vi "Run.vi"(8 "error in (no error)":errorcluster, 11 "C37.118 Sim in":refnum<class "C37.118 Sim.lvclass">) -> (0 "error out":errorcluster, 1 "DataValid":bool, 2 "clSensorData":T1, 3 "C37.118 Sim out":refnum<class "C37.118 Sim.lvclass">)   [LabVIEW 2018, in "SensorPlugins.lvlib" / "C37.118 Sim.lvclass"]
uses:
  C37.118 Sim.lvclass
  C:/projects/ICDAS/NistPluggableModules/Sensor/SensorPlugins/PmuBaseClass/PmuBase.lvclass
  SensorShared/clSensorData.ctl
  PmuBaseClass/PmuBase.lvclass/PmuBase.ctl
  PmuBaseClass/Accessors/Read PmuDataArray.vi
  PmuBaseClass/Accessors/Read PmuConfig.vi
  PmuBaseClass/Accessors/Write PmuDataArray.vi
  SensorShared/SensorShared.lvlib
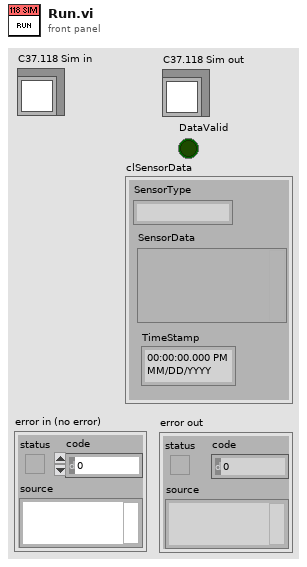
[diagram p1: front panel]
types:
  T1 = typedef "SensorShared.lvlib/clSensorData.ctl" = cluster{"SensorType":string, "SensorData":variant, "TimeStamp":timestamp}
  T2 = typedef "SensorPlugins.lvlib/PmuBase.lvclass/PmuData.ctl" = cluster{"Timestamp":dbl, "Synx":cdb[], "Freq":dbl, "ROCOF":dbl, "ID":i16}
  T3 = typedef "SensorPlugins.lvlib/PmuBase.lvclass/PmuConfig.ctl" = cluster{"Class":enum16{"M", "P"}, "Fs":i32, "F0":i32, "FSamp":i32, "SettlingTime":dbl, "T0":ext}
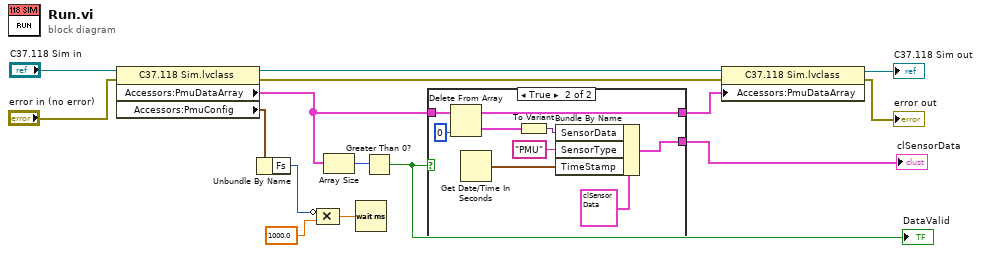
[diagram p0: block diagram]
diagram:
  n1 = property class="C37.118 Sim.lvclass"(reference="C37.118 Sim in", error in="error in (no error)") -> (reference out=w12:refnum<class "C37.118 Sim.lvclass">, error out=w11:errorcluster, "Accessors:PmuDataArray"=w5:T2[], "Accessors:PmuConfig"=w2:T3)
  n2 = Unbundle By Name(w2) -> ("Fs"=w1:i32)
  n3 = Compound Arithmetic op=MULTIPLY(invert w1, 1000.0 ("y")) -> (w8:dbl)
  n4 = Array Size(array=w5) -> (size(s)=w4:i32)
  n5 = Wait (ms)(milliseconds to wait=w8) -> ()  [unwired: 1 out]
  n6 = Greater Than 0?(x=w4) -> (x > 0?=w3:bool)
  "DataValid" <- w3
  n7 = case shown="True" w3 {
    tunnel: [_ w25] -> w9
    tunnel: [w16 w20] -> w6
    tunnel: w5 -> [w16 w18]
    frame False {
    }
    frame True {
      n8 = Delete From Array(array=w18, index=0) -> (deleted portion=w21:T2, array with subset deleted=w20:T2[])  [unwired: 1 in]
      n9 = Get Date/Time In Seconds() -> (seconds since 1Jan1904=w17:timestamp)
      n10 = To Variant(anything=w21) -> (Variant=w23:variant)
      n11 = Bundle By Name(cluster=T1 {"SensorType"="", "SensorData"=variant, "TimeStamp"=timestamp(0 s since 1904-01-01)} ("clSensorData"), "SensorData"=w23, "SensorType"="PMU", "TimeStamp"=w17) -> (w25:T1)
    }
  }
  "clSensorData" <- w9
  n12 = property class="C37.118 Sim.lvclass"(reference=w12, error in=w11, "Accessors:PmuDataArray"=w6) -> (reference out=→"C37.118 Sim out":refnum<class "C37.118 Sim.lvclass">, error out=→"error out":errorcluster)
